vi "test_TrajectoryMG100122AODFrameScan.vi"() -> ()   [LabVIEW 2010, in "TrajectoryMG100122AODFrameScan.lvclass"]
uses:
  TrajectoryMG100122AODFrameScan.lvclass
  common/classes/ErrorController/ErrorController/ErrorController.lvclass
  FPGAWrapper/GenericFPGAWrapper/GenericFPGAWrapper/GenericFPGAWrapper.lvclass
  common/classes/ErrorController/ErrorController/class_data.vi
  common/classes/SpaceVector/SpaceVector/SpaceVector.lvclass
panel:
  out "error handler loaded?":bool
  in  "number of frames":i32
  in  "x angle":dbl[unit](slide) caption="x angle \n(tilting angle, psi)"
  in  "offset z":dbl[unit](slide) scale=0.0..10.0
  in  "offset y":dbl[unit](slide) scale=0.0..10.0
  in  "offset x":dbl[unit](slide) scale=0.0..10.0
  in  "z angle":dbl[unit](slide) caption="z angle \n(rotation angle, phi)"
  in  "zoom":dbl(slide)=1.0 min=1.0 scale=1.0..10.0
  in  "startButton":bool
  in  "createButton":bool
  in  "pixel dwell time":dbl[unit]=9.999999999999999e-06
  in  "stop":bool
  in  "x resolution":i32=256
  in  "y resolution":i32=256
  # "Test VI for TrajectoryMG100122AODFrameScan"
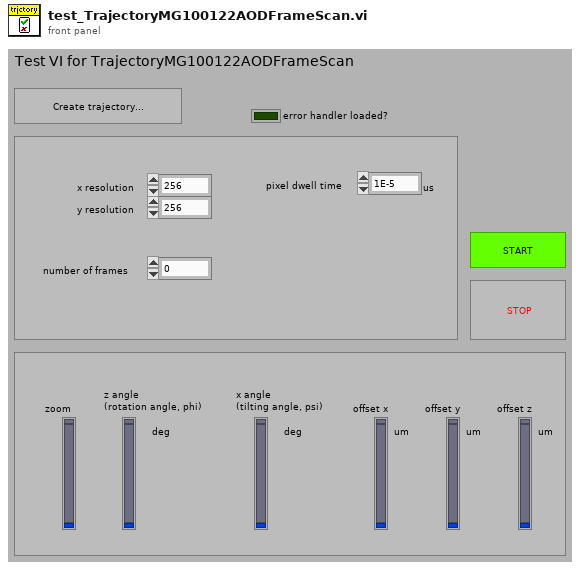
[diagram p1: front panel]
types:
  T1 = typedef "plugin_specification.ctl" = cluster{"class path":string, "configuration":string, "label":string, "settings name":string}
  T2 = typedef "XComponentSpecification.xctl/data.ctl" = cluster{"class path":string, "configuration":string, "label":string, "settings name":string}
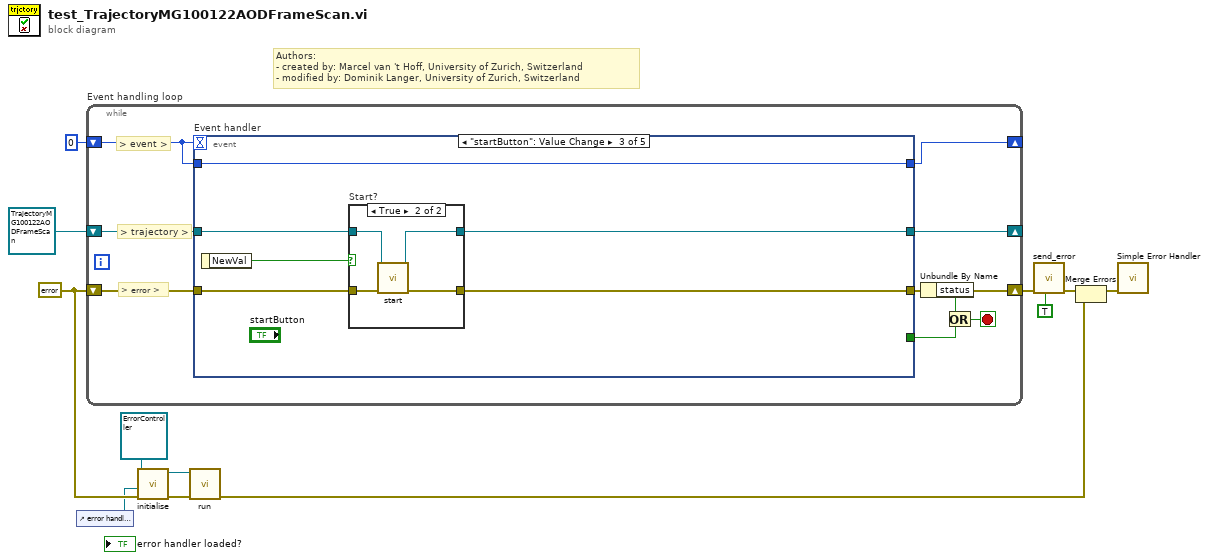
[diagram p0: block diagram]
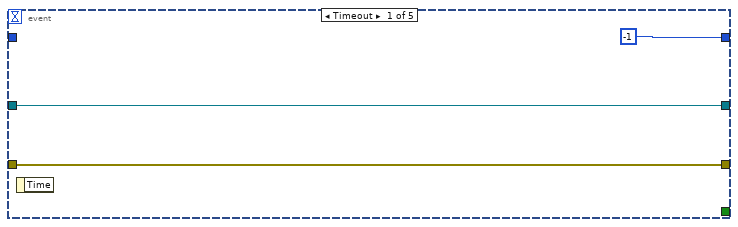
[diagram p2: hidden frame]
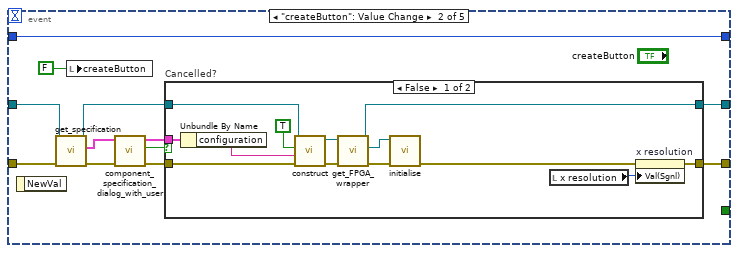
[diagram p3: hidden frame]
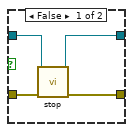
[diagram p5: hidden frame]
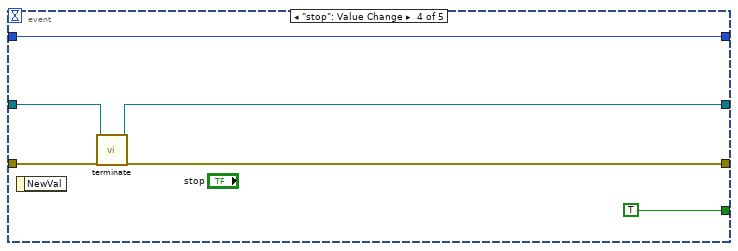
[diagram p6: hidden frame]
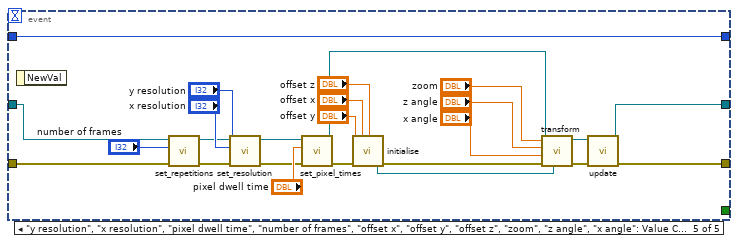
[diagram p7: hidden frame]
diagram:
  w5 = errorcluster {"status"=FALSE, "code"=0, "source"=""} ("error out")
  # "Authors: \n- created by: Marcel van 't Hoff, University of Zurich, Switzerland\n- modified by: Dominik Langer, University of Zurich, Switzerland"
  n1 = control-ref of="error handler loaded?"() -> (w1:refnum<vi>)
  n2 = while "Event handling loop" {
    shift-right: [w14] -> _
    shift-left: 0 -> [w13]
    shift-right: [w18] -> w10
    shift-left: w5 -> [w21]
    shift-right: [w19] -> _
    shift-left: refnum<class "TrajectoryMG100122AODFrameScan.lvclass"> refnum ("TrajectoryMG100122AODFrameScan.lvclass") -> [w20]
    stop <- w16 stop-if-true
    # "> trajectory >"
    # "> error >"
    # "> event >"
    n3 = event "Event handler" shown="[2] \"startButton\": Value Change" {
      selector: _ -> [_ _ _ _ _]
      dyn-events: _ -> [_ _ _ _ _]
      timeout: w13 -> [_ _ _ _ _]
      tunnel: [-1 w36 w57 w70 w96] -> w14
      tunnel: w13 -> [_ w36 w57 w70 w96]
      tunnel: [w22 w33 w54 w68 w78] -> w18
      tunnel: w21 -> [w22 w28 w55 w69 w91]
      tunnel: [w23 w34 w53 w66 w77] -> w19
      tunnel: w20 -> [w23 w30 w56 w67 w89]
      tunnel: [_ _ _ TRUE ("stop") _] -> w15
      event Timeout {
        n4 = event-data() -> ()  [unwired: 1 in, 1 out]
      }
      event "createButton": Value Change {
        n5 = event-data() -> ()  [unwired: 1 in, 1 out]
        n6 = call-dynamic "get_specification.vi"("error in (no error)"=w28, "GenericPlugin in"=w30) -> ("error out"=w27:errorcluster, "component specification"=w31:T1, "GenericPlugin out"=w29:refnum<class "TrajectoryMG100122AODFrameScan.lvclass">)  [unwired: 6 in, 1 out]
        n7 = local write "createButton"(FALSE ("createButton")) -> ()
        n8 = call "component_specification_dialog_with_user.vi"("error in (no error)"=w27, "component specification in"=w31) -> ("error out"=w32:errorcluster, "cancelled?"=w26:bool, "component specification out"=w25:T2)  [unwired: 7 in]
        n9 = case "Cancelled?" shown="False" w26 {
          tunnel: [w40 w51] -> w34
          tunnel: [w48 w50] -> w33
          tunnel: w32 -> [w47 w50]
          tunnel: w29 -> [w46 w51]
          tunnel: w25 -> [w45 _]
          frame False {
            n10 = Unbundle By Name(w45) -> ("configuration"=w44:string)
            n11 = call-dynamic "construct.vi"("error in (no error)"=w47, "configuration name"=w44, "load config file?"=TRUE, "GenericPlugin in"=w46) -> ("error out"=w39:errorcluster, "GenericPlugin out"=w41:refnum<class "TrajectoryMG100122AODFrameScan.lvclass">)  [unwired: 6 in]
            n12 = call-dynamic "get_FPGA_wrapper.vi"("error in (no error)"=w39, "TrajectoryMG100122GenericFPGA in"=w41) -> ("error out"=w38:errorcluster, "GenericFPGAWrapper.lvclass"=w42:refnum<class "GenericFPGAWrapper.lvclass">, "TrajectoryMG100122GenericFPGA out"=w40:refnum<class "TrajectoryMG100122AODFrameScan.lvclass">)  [unwired: 7 in]
            n13 = call-dynamic "initialise.vi"("error in (no error)"=w38, "GenericPlugin in"=w42) -> ("error out"=w37:errorcluster)  [unwired: 8 in, 1 out]
            n14 = local read "x resolution"() -> (w49:i32)
            n15 = property on="x resolution" class="DigNum (strict)"(error in=w37, "Val(Sgnl)"=w49) -> (error out=w48:errorcluster)  [unwired: 1 in, 1 out]
          }
          frame True {
          }
        }
      }
      event "startButton": Value Change {
        n16 = event-data() -> ("NewVal"=w52:bool)  [unwired: 1 in]
        n17 = case "Start?" shown="True" w52 {
          tunnel: w56 -> [w59 w65]
          tunnel: w55 -> [w61 w64]
          tunnel: [w60 w63] -> w54
          tunnel: [w58 w62] -> w53
          frame False {
            n18 = call-dynamic "stop.vi"("error in (no error)"=w61, "TrajectoryMG100122GenericFPGA in"=w59) -> ("error out"=w60:errorcluster, "TrajectoryMG100122GenericFPGA out"=w58:refnum<class "TrajectoryMG100122AODFrameScan.lvclass">)  [unwired: 8 in]
          }
          frame True {
            n19 = call-dynamic "start.vi"("error in (no error)"=w64, "TrajectoryMG100122GenericFPGA in"=w65) -> ("error out"=w63:errorcluster, "TrajectoryMG100122GenericFPGA out"=w62:refnum<class "TrajectoryMG100122AODFrameScan.lvclass">)  [unwired: 8 in]
          }
        }
      }
      event "stop": Value Change {
        n20 = event-data() -> ()  [unwired: 1 in, 1 out]
        n21 = call-dynamic "terminate.vi"("error in (no error)"=w69, "GenericPlugin in"=w67) -> ("error out"=w68:errorcluster, "GenericPlugin out"=w66:refnum<class "TrajectoryMG100122AODFrameScan.lvclass">)  [unwired: 8 in]
      }
      event "y resolution", "x resolution", "pixel dwell time", "number of frames", "offset x", "offset y", "offset z", "zoom", "z angle", "x angle": Value Change {
        n22 = event-data() -> ()  [unwired: 1 in, 1 out]
        n23 = call-dynamic "set_repetitions.vi"("error in (no error)"=w91, "repetitions"="number of frames", "GenericTrajectory in"=w89) -> ("error out"=w90:errorcluster, "GenericTrajectory out"=w88:refnum<class "TrajectoryMG100122AODFrameScan.lvclass">)  [unwired: 7 in]
        n24 = call-dynamic "set_resolution.vi"("error in (no error)"=w90, "y resolution"="y resolution", "x resolution"="x resolution", "TrajectoryMG100122AODFrameScan in"=w88) -> ("error out"=w75:errorcluster, "TrajectoryMG100122AODFrameScan out"=w74:refnum<class "TrajectoryMG100122AODFrameScan.lvclass">)  [unwired: 6 in]
        n25 = call-dynamic "set_pixel_times.vi"("error in (no error)"=w75, "pixel dwell time"="pixel dwell time", "TrajectoryMG100122AODFrameScan in"=w74) -> ("error out"=w76:errorcluster, "TrajectoryMG100122AODFrameScan out"=w79:refnum<class "TrajectoryMG100122AODFrameScan.lvclass">)  [unwired: 7 in]
        n26 = call "initialise.vi"("z"="offset z", "error in (no error)"=w76, "y"="offset y", "x"="offset x") -> ("error out"=w85:errorcluster, "SpaceVector out"=w81:refnum<class "SpaceVector.lvclass">)  [unwired: 6 in]
        n27 = call-dynamic "transform.vi"("SpaceVector.lvclass"=w81, "zoom"="zoom", "error in (no error)"=w85, "x angle (psi)"="x angle", "z angle (phi)"="z angle", "TrajectoryMG100122AODFrameScan in"=w79) -> ("error out"=w72:errorcluster, "TrajectoryMG100122AODFrameScan out"=w73:refnum<class "TrajectoryMG100122AODFrameScan.lvclass">)  [unwired: 4 in]
        n28 = call-dynamic "update.vi"("error in (no error)"=w72, "TrajectoryMG100122AODFrameScan in"=w73) -> ("error out"=w78:errorcluster, "TrajectoryMG100122AODFrameScan out"=w77:refnum<class "TrajectoryMG100122AODFrameScan.lvclass">)  [unwired: 8 in]
      }
    }
    n29 = Unbundle By Name(w18) -> ("status"=w17:bool)
    n30 = Or(x=w17, y=w15) -> (x .or. y?=w16:bool)
  }
  n31 = call-dynamic "initialise.vi"("error in (no error)"=w5, "error boolean"=w1, "ErrorController in"=refnum<class "ErrorController.lvclass"> refnum ("ErrorController.lvclass")) -> ("error out"=w4:errorcluster, "ErrorController out"=w2:refnum<class "ErrorController.lvclass">)  [unwired: 7 in]
  n32 = call "run.vi"("error in (no error)"=w4, "ErrorController in"=w2) -> ("error out"=w7:errorcluster)  [unwired: 8 in, 1 out]
  n33 = call "send_error.vi"("last error? (F)"=TRUE, "error in (no error)"=w10) -> ("error out"=w8:errorcluster)  [unwired: 9 in]
  n34 = Merge Errors(w8, w7) -> (w6:errorcluster)
  n35 = call <vilib>:"Simple Error Handler.vi"("error in (no error)"=w6) -> ()  [unwired: 4 in, 5 out]
